vi "NovRAM Dump.vi"() -> ()   [LabVIEW 2009, in "Digikrom DK24x.lvlib"]
doc: "Reads current NOVRAM contents and saves it to a file."
uses:
  Digikrom DK24x.lvlib
panel:
  in  "VISA resource name":refnum<visa-resource-name>="COM1"
  out "NoVRam Dump":string
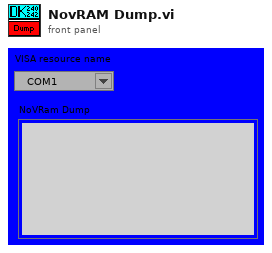
[diagram p1: front panel]
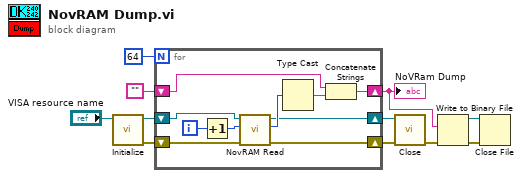
[diagram p0: block diagram]
diagram:
  n1 = call "Initialize.vi"("VISA resource name"="VISA resource name") -> ("error out"=w10:errorcluster, "VISA resource name out"=w9:refnum<visa-resource-name>)  [unwired: 1 in, 8 out]
  n2 = for {
    N: 64 -> [_]
    shift-right: [w13] -> w4
    shift-left: w10 -> [w17]
    shift-right: [w14] -> w3
    shift-left: w9 -> [w18]
    shift-right: [w19] -> w1
    shift-left: "" -> [w21]
    i -> [w16]
    n3 = Increment(x=w16) -> (x+1=w12:i32)
    n4 = call "NovRAM Read.vi"("error in (no error)"=w17, "NOVRAM ADDRESS"=w12, "VISA resource name"=w18) -> ("error out"=w13:errorcluster, "WORD READ"=w15:u16, "VISA resource name out"=w14:refnum<visa-resource-name>)  [unwired: 6 out]
    n5 = Type Cast(x=w15) -> (*(type *) &x=w20:string)  [unwired: 1 out]
    n6 = Concatenate Strings(w21, w20) -> (w19:string)
  }
  "NoVRam Dump" <- w1
  n7 = call "Close.vi"("error in (no error)"=w4, "VISA resource name"=w3) -> ("error out"=w2:errorcluster)  [unwired: 9 out]
  n8 = Write to Binary File(data=w1, error in=w2) -> (refnum out=w5:refnum<file>, error out=w6:errorcluster)  [unwired: 5 out]
  n9 = Close File(refnum=w5, error in=w6) -> ()  [unwired: 2 out]
